vi "HEWH Extract End of Draw Data.vi"(4 "Draw Start":i32, 6 "Program Status Index":i32, 7 "Test Data-Start to End DBL":dbl[][](array[numeric]), 8 "error in (no error)":errorcluster, 9 "Test Data -Start to End (String)":string[][](array[string]), 10 "Flow Rate Index":i32, 11 "Heat Source Index":i32) -> (0 "error out":errorcluster, 1 "Program Status":string[](array[string]), 3 "Totalized Flow":dbl[](array[numeric]), 5 "Flow Rate":dbl[](array[numeric]))   [LabVIEW 2023]
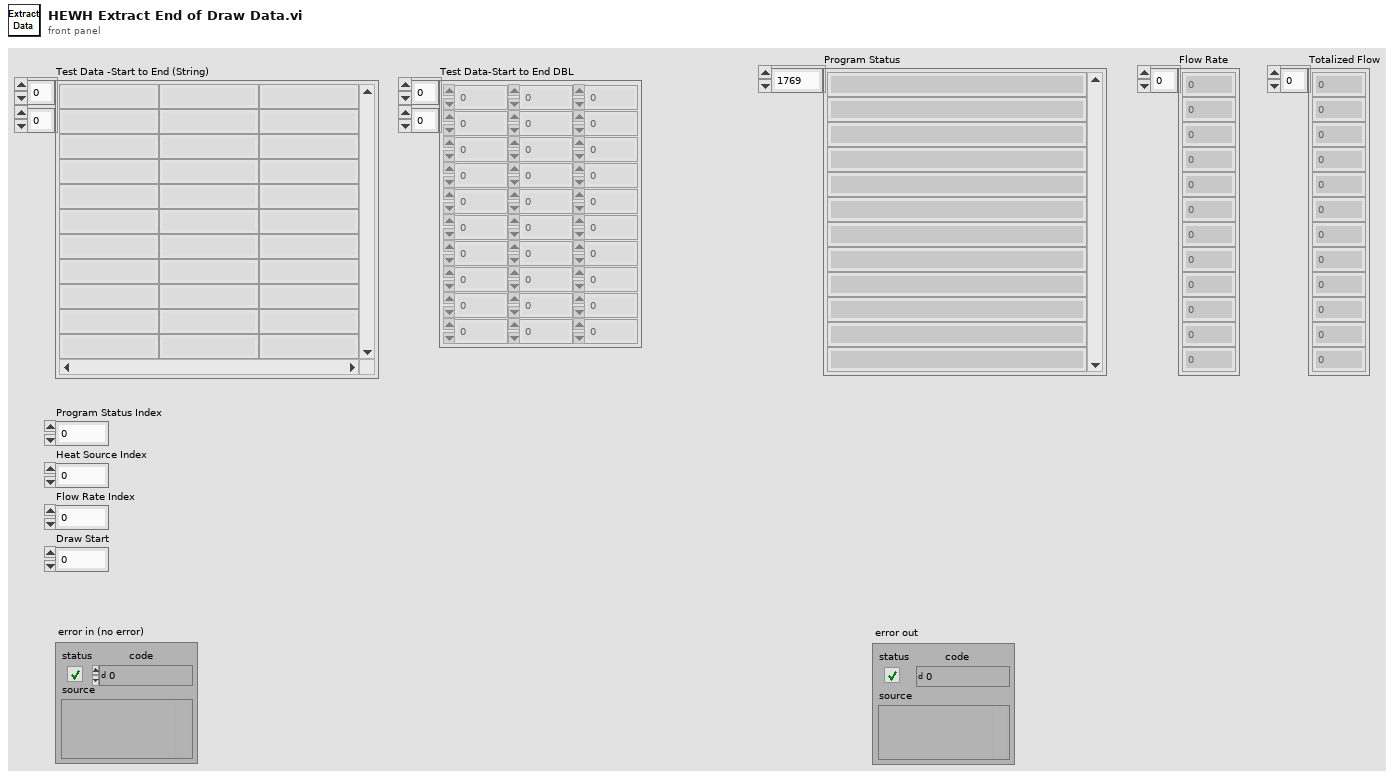
[diagram p1: front panel]
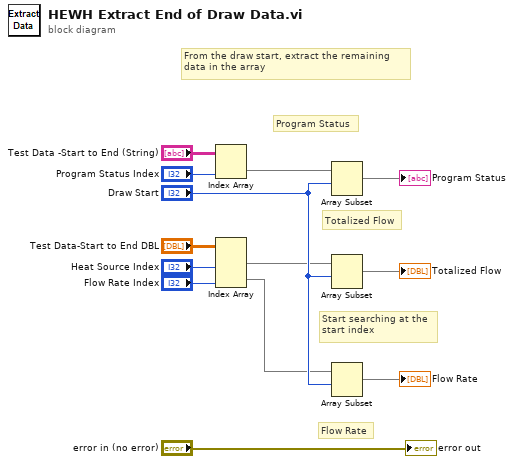
[diagram p0: block diagram]
diagram:
  # "From the draw start, extract the remaining \ndata in the array"
  # "Program Status"
  # "Flow Rate"
  # "Totalized Flow"
  # "Start searching at the \nstart index"
  n1 = Index Array(array="Test Data -Start to End (String)", index (col)="Program Status Index") -> (element=w10:string[])  [unwired: 1 in]
  n2 = Index Array(array="Test Data-Start to End DBL", index (col) #1="Heat Source Index", index (col) #2="Flow Rate Index") -> (element #1=w2:dbl[], element #2=w4:dbl[])  [unwired: 2 in]
  n3 = Array Subset(array=w10, index="Draw Start") -> (→"Program Status":string[])  [unwired: 1 in]
  n4 = Array Subset(array=w2, index="Draw Start") -> (→"Totalized Flow":dbl[])  [unwired: 1 in]
  n5 = Array Subset(array=w4, index="Draw Start") -> (→"Flow Rate":dbl[])  [unwired: 1 in]
  "error out" <- "error in (no error)"
